vi "Translation3d_Equals.vi"(9 "other Translation3d":T1 {"Z" format="%14.3f"; "Y" format="%14.3f"; "X" format="%14.3f"}, 11 "In Translation3d":T1 {"Z" format="%14.3f"; "Y" format="%14.3f"; "X" format="%14.3f"}) -> (3 "Equals":bool)   [LabVIEW 2019, in "Trajectory_Library.lvlib"]
doc: "Checks equality between this Translation2d and another object.\n\nParameters:\n - IN TRANSLATION - This TRANSLATION data structure\n - OTHER TRANSLATION - The other TRANSLATION data structure\n\nReturns:\n - EQUALS - Value is set to TRUE if the two TRANSLATIONS are equal."
uses:
  Trajectory_Library.lvlib
  TRANSLATION3D.ctl
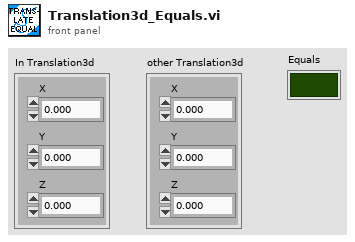
[diagram p1: front panel]
types:
  T1 = typedef "Trajectory_Library.lvlib/TRANSLATION3D.ctl" = cluster{"X":dbl, "Y":dbl, "Z":dbl}
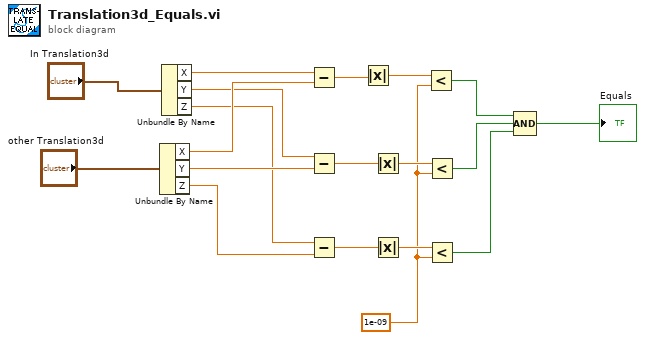
[diagram p0: block diagram]
diagram:
  w4 = 1e-09 ("y")
  n1 = Unbundle By Name("other Translation3d") -> ("X"=w16:dbl, "Y"=w15:dbl, "Z"=w2:dbl)
  n2 = Unbundle By Name("In Translation3d") -> ("X"=w17:dbl, "Y"=w14:dbl, "Z"=w3:dbl)
  n3 = Subtract(x=w17, y=w16) -> (x-y=w12:dbl)
  n4 = Subtract(x=w14, y=w15) -> (x-y=w13:dbl)
  n5 = Subtract(x=w3, y=w2) -> (x-y=w6:dbl)
  n6 = Absolute Value(x=w12) -> (abs(x)=w10:dbl)
  n7 = Absolute Value(x=w13) -> (abs(x)=w11:dbl)
  n8 = Absolute Value(x=w6) -> (abs(x)=w5:dbl)
  n9 = Less?(x=w10, y=w4) -> (x < y?=w9:bool)
  n10 = Less?(x=w11, y=w4) -> (x < y?=w8:bool)
  n11 = Less?(x=w5, y=w4) -> (x < y?=w1:bool)
  n12 = Compound Arithmetic op=AND(w9, w8, w1) -> (→"Equals":bool)
